vi "Begin.vi"() -> (0 "error out":errorcluster)   [LabVIEW 2013]
doc: "Called before other user functions, this VI is expected to open initial I/O refnums, load in file data, and do all program initialization. Notice that the <B>error out</B> terminal is simply used for data flow. Wiring it to other structures or subVIs ensures that this VI runs first."
uses:
  <vilib>/Rock Robotics/WPI/Joystick/WPI_JoystickDeviceEnum.ctl
  <vilib>/Rock Robotics/SystemInterfaces/Typedef/FPGA_TypedefDigitalModule.ctl
  <vilib>/Rock Robotics/SystemInterfaces/DIO/FPGA_DIOChannel.ctl
  <vilib>/Rock Robotics/SystemInterfaces/DIO/FPGA_DIORelayChannel.ctl
  <vilib>/Rock Robotics/SystemInterfaces/Typedef/FPGA_TypedefSolenoidModule.ctl
  <vilib>/Rock Robotics/WPI/Solenoid/WPI_SolenoidChannel.ctl
  <vilib>/Rock Robotics/WPI/Solenoid/WPI_SolenoidValue.ctl
  <vilib>/Rock Robotics/SystemInterfaces/DIO/FPGA_DIOPWMChannel.ctl
  <vilib>/Rock Robotics/WPI/Encoder/WPI_EncoderType.ctl
  <vilib>/Rock Robotics/WPI/Solenoid/WPI_SolenoidOpenDouble.vi
  <vilib>/Rock Robotics/WPI/Solenoid/WPI_SolenoidSetEnum.vi
  <vilib>/Rock Robotics/WPI/Counter/WPI_CounterDigitalInputToDigitalSource.vi
  <vilib>/Rock Robotics/WPI/RobotDrive/WPI_RobotDriveOpen2MotorWithVictor.vi
  <vilib>/Rock Robotics/WPI/MotorControl/WPI_MotorControlOpen Victor.vi
  <vilib>/Rock Robotics/WPI/Compressor/WPI_CompressorGetSetRefNum.vi
  <vilib>/Rock Robotics/WPI/Camera/WPI_CameraImageSize.ctl
  <vilib>/Rock Robotics/WPI/Camera/WPI_CameraWhite Balance Values.ctl
  <vilib>/Rock Robotics/WPI/Camera/WPI_CameraExposure Values.ctl
  <vilib>/Rock Robotics/WPI/Camera/WPI_CameraFrameRate.ctl
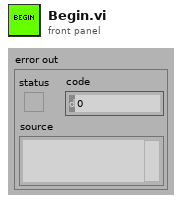
[diagram p1: front panel]
types:
  T1 = typedef "FPGA_DIOChannel.ctl" = enum8{"DIO 1", "DIO 2", "DIO 3", "DIO 4", "DIO 5", "DIO 6", "DIO 7", "DIO 8", "DIO 9", "DIO 10", "DIO 11", "DIO 12", "DIO 13", "DIO 14", "Invalid"}
  T2 = typedef "WPI_SolenoidChannel.ctl" = enum8{"Solenoid 1", "Solenoid 2", "Solenoid 3", "Solenoid 4", "Solenoid 5", "Solenoid 6", "Solenoid 7", "Solenoid 8", "Invalid"}
  T3 = typedef "FPGA_DIOPWMChannel.ctl" = enum8{"PWM 1", "PWM 2", "PWM 3", "PWM 4", "PWM 5", "PWM 6", "PWM 7", "PWM 8", "PWM 9", "PWM 10", "Invalid"}
  T4 = typedef "WPI_EncoderType.ctl" = enum16{"1x", "2x", "4x"}
  T5 = typedef "WPI_SolenoidValue.ctl" = enum16{"Off", "On", "Forward", "Reverse"}
  T6 = typedef "FPGA_TypedefSolenoidModule.ctl" = enum16{"Solenoid Module 1", "Solenoid Module 2"}
  T7 = typedef "FPGA_DIORelayChannel.ctl" = enum8{"Relay 1", "Relay 2", "Relay 3", "Relay 4", "Relay 5", "Relay 6", "Relay 7", "Relay 8", "Invalid"}
  T8 = typedef "WPI_JoystickDeviceEnum.ctl" = enum16{"USB 1", "USB 2", "USB 3", "USB 4", "Kinect 1", "Kinect 2"}
  T9 = typedef "FPGA_TypedefDigitalModule.ctl" = enum16{"Digital Module 1", "Digital Module 2"}
  T10 = typedef "WPI_CameraFrameRate.ctl" = u32
  T11 = typedef "WPI_CameraExposure Values.ctl" = enum16{"Auto", "Flicker-free 50 Hz", "Flicker-free 60 Hz", "Hold current"}
  T12 = typedef "WPI_CameraWhite Balance Values.ctl" = enum16{"Auto", "Fixed indoor", "Fixed outdoor 1", "Fixed outdoor 2", "Fixed fluorescent 1", "Fixed fluorescent 2", "Hold current"}
  T13 = typedef "WPI_CameraImageSize.ctl" = enum16{"640x480", "320x240", "160x120"}
  T14 = typedef "WPI_CameraDevRef.ctl" = cluster{"Camera Address":string, "CameraStatus":errorcluster, "Acquire Image Notifier":refnum<notifier>}
  T15 = typedef "WPI_DigitalInputDevRef.ctl" = cluster{"DevStatus":errorcluster, "DIO Channel":T1, "Digital Module":T9}
  T16 = typedef "WPI_MotorControlDeviceRef.ctl" = cluster{"DeviceStatus":errorcluster, "Type":enum16{"PWM", "CAN"}, "PWM":cluster{"Digital Module":T9, "PWM Channel":T3, "DeadBand":T17}, "CAN":cluster{"Device Number":u8, "Control Mode":T18, "Semaphore":T19, "Max Vout":dbl}, "Invert":bool, "TransformRef":T20, "InvTransformRef":T20}
  T17 = typedef "WPI_PWMDeadband.ctl" = cluster{"Name":string, "maxPositivePwm":i32, "minPositivePwm":i32, "centerPwm":i32, "maxNegativePwm":i32, "minNegativePwm":i32, "angularRange":u16}
  T18 = typedef "WPI_CANJaguar_ControlMode.ctl" = enum8{"Percent VBus", "Current", "Speed", "Position", "Voltage"}
  T19 = typedef "Semaphore RefNum" = refnum<k1>
  T20 = typedef "WPI_PWMTransform_ConPane.ctl" = refnum<vi>
  T21 = typedef "WPI_SolenoidDevRef.ctl" = cluster{"DevStatus":errorcluster, "Solenoid Module":T6, "Forward Solenoid Channel":T2, "Reverse Solenoid Channel":T2}
  T22 = typedef "FPGA_CounterEncoderSourceConvertionLVSourceType.ctl" = cluster{"DevStatus":errorcluster, "AnalogTriggerMode?":bool, "DigitalMode":cluster{"Digital Module":T9, "DIO Channel":T23}, "AnalogTriggerMode":cluster{"AnalogTriggerIndex":T24, "OutputType":T25}}
  T23 = typedef "FPGA_DIODigitalSourceChannel.ctl" = enum8{"DIO 1", "DIO 2", "DIO 3", "DIO 4", "DIO 5", "DIO 6", "DIO 7", "DIO 8", "DIO 9", "DIO 10", "DIO 11", "DIO 12", "DIO 13", "DIO 14", "Disabled"}
  T24 = typedef "FPGA_AnalogTriggerIndex.ctl" = enum8{"Trig 0", "Trig 1", "Trig 2", "Trig 3", "Trig 4", "Trig 5", "Trig 6", "Trig 7", "Invalid"}
  T25 = typedef "FPGA_AnalogTriggerOutType.ctl" = enum16{"InWindow", "TriggerState", "Rising", "Falling"}
  T26 = typedef "WPI_CompressorDevRef.ctl" = cluster{"DevStatus":errorcluster, "DigitalInputDevRef":T15, "RelayDevRef":T27}
  T27 = typedef "WPI_RelayDevRef.ctl" = cluster{"DevStatus":errorcluster, "Relay Channel":T7, "Digital Module":T9, "Relay Direction":T28}
  T28 = typedef "WPI_RelayDirection.ctl" = enum16{"Both directions", "Forward only", "Reverse only"}
  T29 = typedef "WPI_RobotDriveDevRef.ctl" = cluster{"DevStatus":errorcluster, "Motors[]":T16[], "Square Inputs":bool, "Max Output":dbl, "Isochronous":bool}
  T30 = typedef "WPI_EncoderDevRef.ctl" = cluster{"DevStatus":errorcluster, "EncoderIndex":T31, "CounterIndex":T32, "DistancePerCount":dbl, "Decoding Type":T4}
  T31 = typedef "FPGA_EncoderIdx.ctl" = enum8{"Enc 0", "Enc 1", "Enc 2", "Enc 3", "Invalid"}
  T32 = typedef "FPGA_CounterCtrSystemIndex.ctl" = enum8{"Ctr 0", "Ctr 1", "Ctr 2", "Ctr 3", "Ctr 4", "Ctr 5", "Ctr 6", "Ctr 7", "Invalid"}
  T33 = typedef "WPI_JoystickDevRef.ctl" = cluster{"Device":T8}
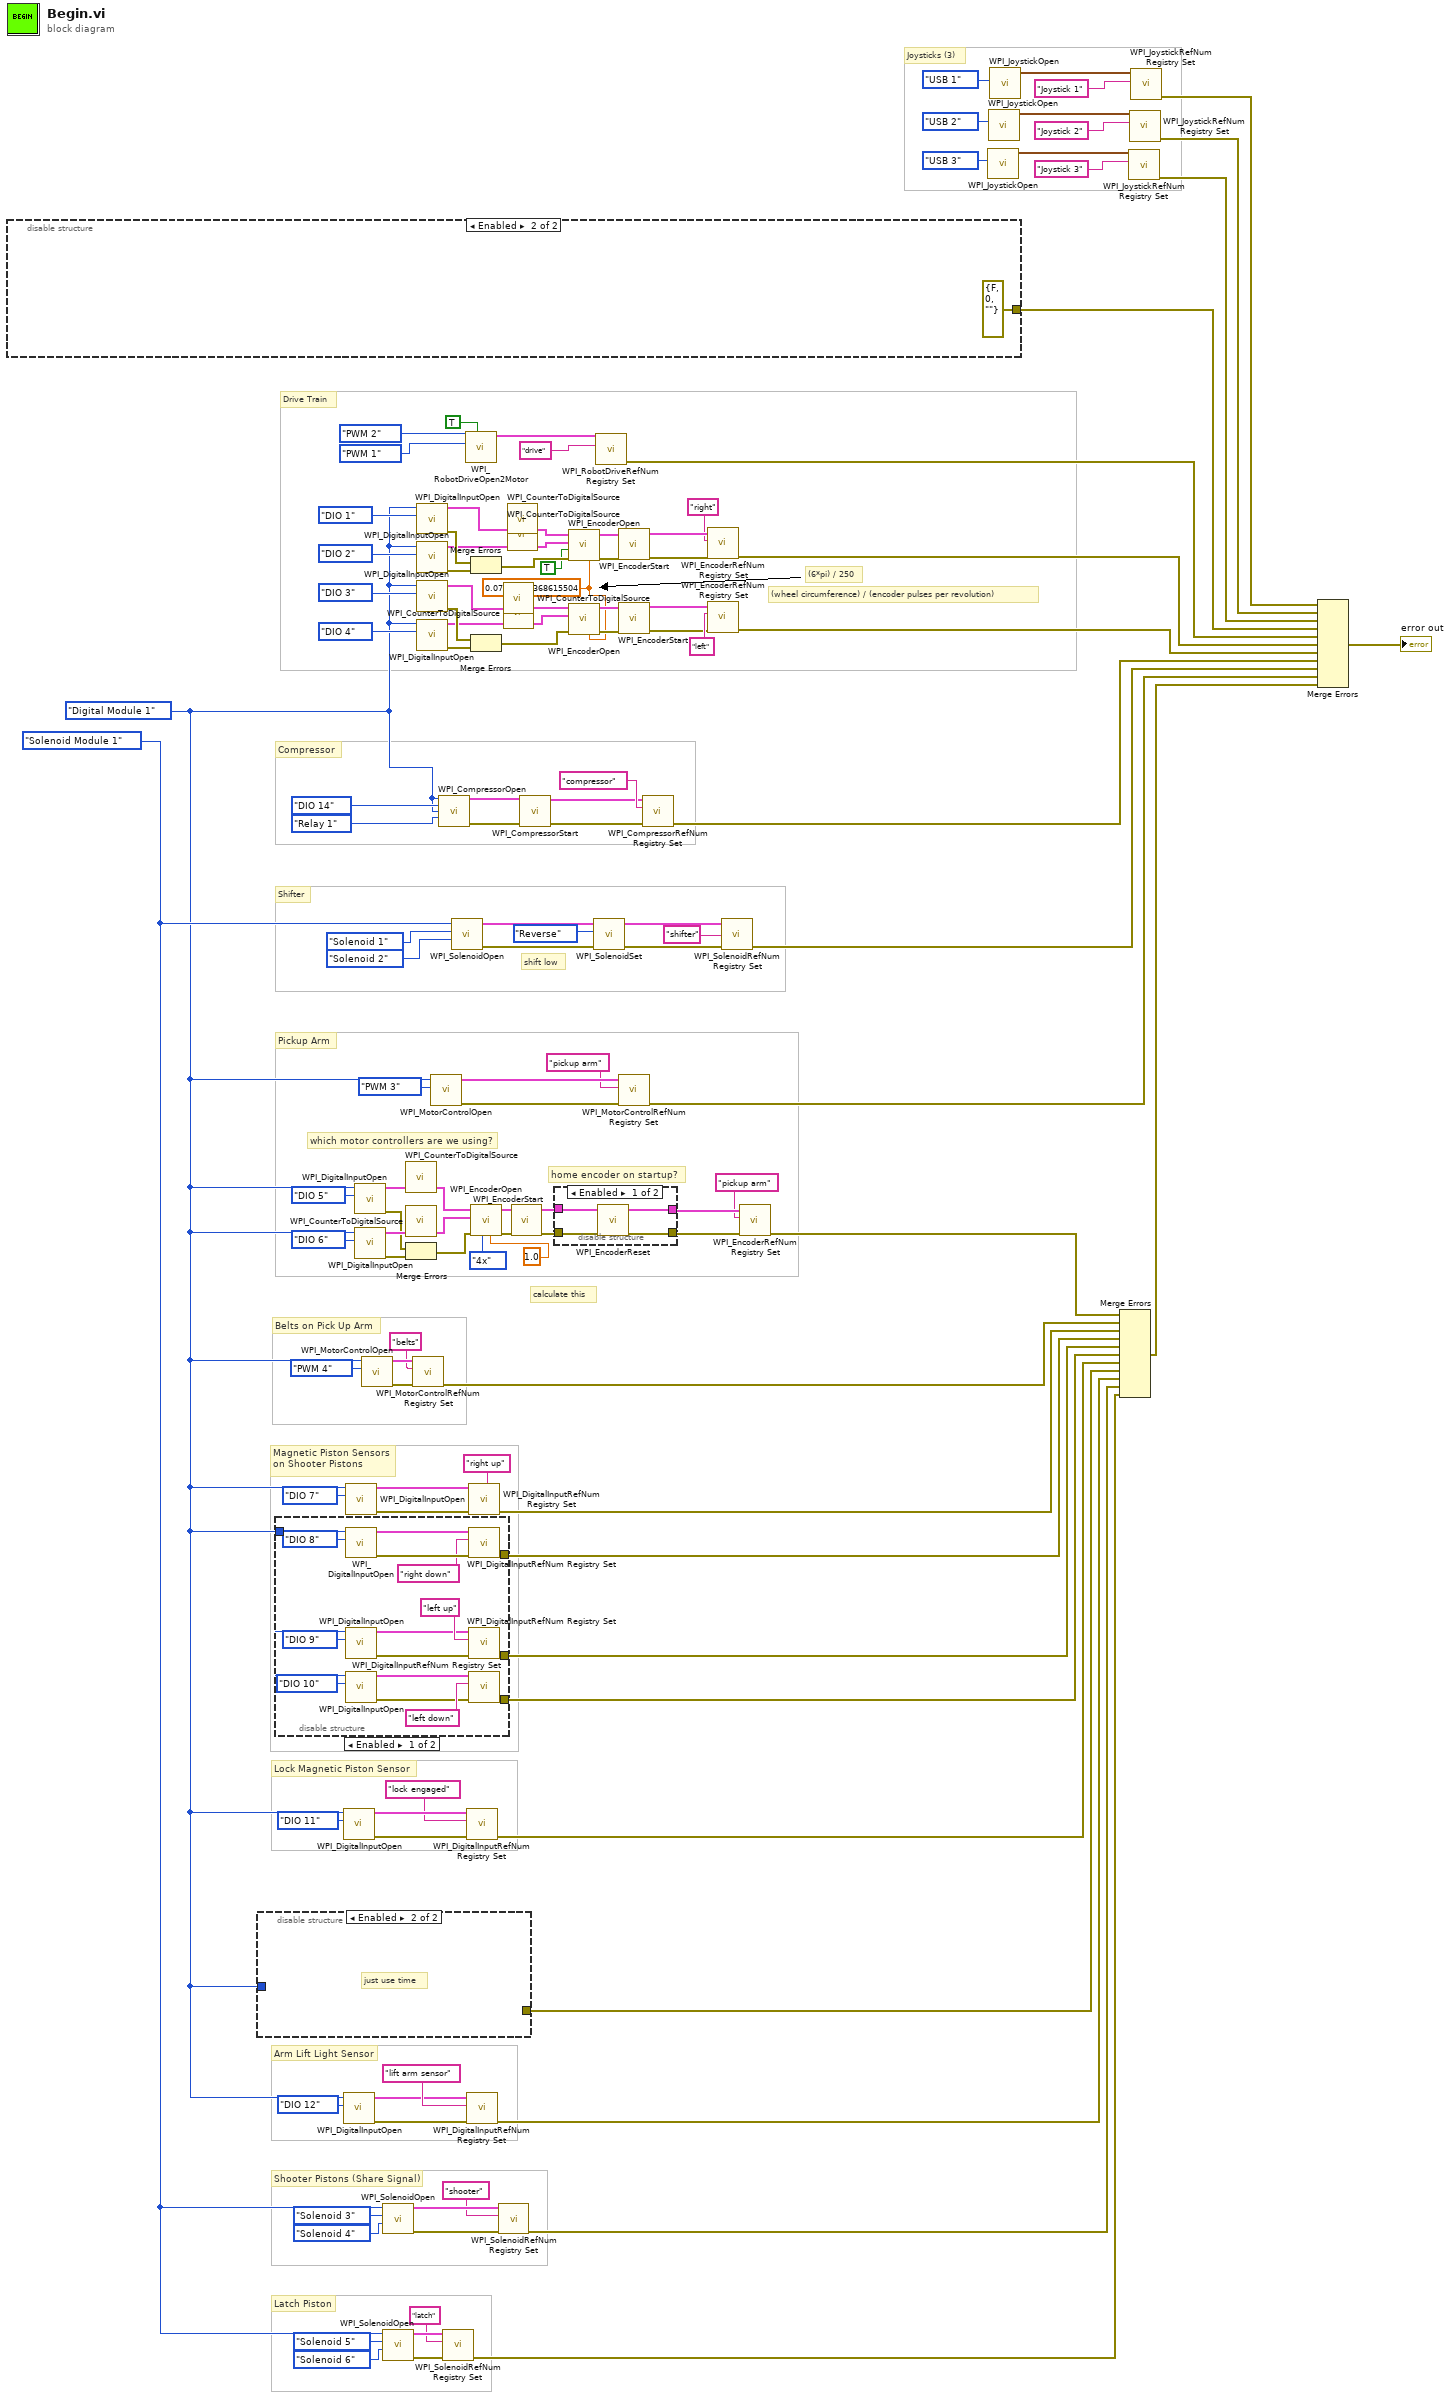
[diagram p0: block diagram]
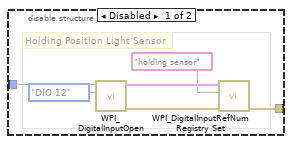
[diagram p3: hidden frame]
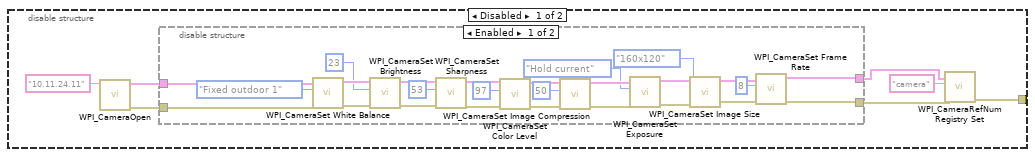
[diagram p5: hidden frame]
diagram:
  w76 = 0.07539822368615504 ("DistancePerCount")
  w17 = FPGA_TypedefSolenoidModule."Solenoid Module 1" ("Solenoid Module (Module 1)")
  w6 = FPGA_TypedefDigitalModule."Digital Module 1" ("Digital Module (Module 1)")
  # "Lock Magnetic Piston Sensor"
  # "Arm Lift Light Sensor"
  # "Joysticks (3)"
  # "Latch Piston"
  # "Shooter Pistons (Share Signal)"
  # "Magnetic Piston Sensors\non Shooter Pistons"
  # "Belts on Pick Up Arm"
  # "calculate this"
  # "Pickup Arm"
  # "home encoder on startup?"
  # "Shifter"
  # "Compressor"
  # "Drive Train"
  # "which motor controllers are we using?"
  # "shift low"
  # "(wheel circumference) / (encoder pulses per revolution)"
  # "(6*pi) / 250"
  n1 = disable-structure shown="Enabled" {
    disable-tunnel: [w133 errorcluster {"status"=FALSE, "code"=0, "source"=""} ("error out")] -> w120
    frame Disabled {
      n2 = call <vilib>:"WPI_CameraOpen.vi"("Camera Address"="10.11.24.11") -> ("error out"=w135:errorcluster, "CameraDevRef"=w137:T14)  [unwired: 9 in]
      n3 = disable-structure shown="Enabled" {
        disable-tunnel: w137 -> [w163 w167]
        disable-tunnel: [w141 w167] -> w136
        disable-tunnel: w135 -> [w150 w166]
        disable-tunnel: [w140 w166] -> w134
        frame Enabled {
          n4 = call <vilib>:"WPI_CameraSet White Balance.vi"("error in (no error)"=w150, "White Balance"=WPI_CameraWhite_Balance_Values."Fixed outdoor 1", "CameraDevRef"=w163) -> ("error out"=w151:errorcluster, "CameraDevRef Out"=w162:T14)  [unwired: 7 in]
          n5 = call <vilib>:"WPI_CameraSet Brightness.vi"("error in (no error)"=w151, "Brightness"=23, "CameraDevRef"=w162) -> ("error out"=w152:errorcluster, "CameraDevRef Out"=w161:T14)  [unwired: 7 in]
          n6 = call <vilib>:"WPI_CameraSet Sharpness.vi"("error in (no error)"=w152, "Sharpness"=53, "CameraDevRef"=w161) -> ("error out"=w153:errorcluster, "CameraDevRef Out"=w160:T14)  [unwired: 7 in]
          n7 = call <vilib>:"WPI_CameraSet Color Level.vi"("error in (no error)"=w153, "Color Level"=97, "CameraDevRef"=w160) -> ("error out"=w154:errorcluster, "CameraDevRef Out"=w159:T14)  [unwired: 7 in]
          n8 = call <vilib>:"WPI_CameraSet Image Compression.vi"("error in (no error)"=w154, "Compression"=50, "CameraDevRef"=w159) -> ("error out"=w165:errorcluster, "CameraDevRef Out"=w164:T14)  [unwired: 7 in]
          n9 = call <vilib>:"WPI_CameraSet Exposure.vi"("error in (no error)"=w165, "Exposure"=WPI_CameraExposure_Values."Hold current", "CameraDevRef"=w164) -> ("error out"=w155:errorcluster, "CameraDevRef Out"=w158:T14)  [unwired: 7 in]
          n10 = call <vilib>:"WPI_CameraSet Image Size.vi"("error in (no error)"=w155, "Image Size"=WPI_CameraImageSize."160x120", "CameraDevRef"=w158) -> ("error out"=w156:errorcluster, "CameraDevRef Out"=w157:T14)  [unwired: 7 in]
          n11 = call <vilib>:"WPI_CameraSet Frame Rate.vi"("error in (no error)"=w156, "Frame Rate (fps)"=T10 8, "CameraDevRef"=w157) -> ("error out"=w140:errorcluster, "CameraDevRef Out"=w141:T14)  [unwired: 7 in]
        }
        frame Disabled {
        }
      }
      n12 = call <vilib>:"WPI_CameraRefNum Registry Set.vi"("error in (no error)"=w134, "refnum name"="camera", "CameraDevRef"=w136) -> ("error out"=w133:errorcluster)  [unwired: 7 in, 1 out]
    }
    frame Enabled {
    }
  }
  n13 = disable-structure shown="Enabled" {
    disable-tunnel: w6 -> [w170 _]
    disable-tunnel: [w169 _] -> w2
    frame Disabled {
      # "Holding Position Light Sensor"
      n14 = call <vilib>:"WPI_DigitalInputOpen.vi"("DIO Channel"=FPGA_DIOChannel."DIO 12", "Digital Module (Module 1)"=w170) -> ("error out"=w173:errorcluster, "DigitalInputDevRef"=w172:T15)  [unwired: 8 in]
      n15 = call <vilib>:"WPI_DigitalInputRefNum Registry Set.vi"("error in (no error)"=w173, "refnum name"="holding sensor", "DigitalInputDevRef"=w172) -> ("error out"=w169:errorcluster)  [unwired: 7 in, 1 out]
    }
    frame Enabled {
      # "just use time"
    }
  }
  n16 = disable-structure shown="Enabled" {
    disable-tunnel: [w187 _] -> w28
    disable-tunnel: w6 -> [w177 _]
    disable-tunnel: [w176 _] -> w12
    disable-tunnel: [w175 _] -> w11
    frame Enabled {
      n17 = call <vilib>:"WPI_DigitalInputOpen.vi"("DIO Channel"=FPGA_DIOChannel."DIO 8", "Digital Module (Module 1)"=w177) -> ("error out"=w190:errorcluster, "DigitalInputDevRef"=w189:T15)  [unwired: 8 in]
      n18 = call <vilib>:"WPI_DigitalInputOpen.vi"("DIO Channel"=FPGA_DIOChannel."DIO 9", "Digital Module (Module 1)"=w177) -> ("error out"=w178:errorcluster, "DigitalInputDevRef"=w179:T15)  [unwired: 8 in]
      n19 = call <vilib>:"WPI_DigitalInputOpen.vi"("DIO Channel"=FPGA_DIOChannel."DIO 10", "Digital Module (Module 1)"=w177) -> ("error out"=w180:errorcluster, "DigitalInputDevRef"=w181:T15)  [unwired: 8 in]
      n20 = call <vilib>:"WPI_DigitalInputRefNum Registry Set.vi"("error in (no error)"=w190, "refnum name"="right down", "DigitalInputDevRef"=w189) -> ("error out"=w187:errorcluster)  [unwired: 7 in, 1 out]
      n21 = call <vilib>:"WPI_DigitalInputRefNum Registry Set.vi"("error in (no error)"=w178, "refnum name"="left up", "DigitalInputDevRef"=w179) -> ("error out"=w176:errorcluster)  [unwired: 7 in, 1 out]
      n22 = call <vilib>:"WPI_DigitalInputRefNum Registry Set.vi"("error in (no error)"=w180, "refnum name"="left down", "DigitalInputDevRef"=w181) -> ("error out"=w175:errorcluster)  [unwired: 7 in, 1 out]
    }
    frame Disabled {
      # "dang, only one sensor\non the pistons..."
    }
  }
  n23 = call <vilib>:"WPI_DigitalInputOpen.vi"("DIO Channel"=FPGA_DIOChannel."DIO 11", "Digital Module (Module 1)"=w6) -> ("error out"=w9:errorcluster, "DigitalInputDevRef"=w8:T15)  [unwired: 8 in]
  n24 = call <vilib>:"WPI_DigitalInputOpen.vi"("DIO Channel"=FPGA_DIOChannel."DIO 12", "Digital Module (Module 1)"=w6) -> ("error out"=w14:errorcluster, "DigitalInputDevRef"=w15:T15)  [unwired: 8 in]
  n25 = call <vilib>:"WPI_DigitalInputOpen.vi"("DIO Channel"=FPGA_DIOChannel."DIO 7", "Digital Module (Module 1)"=w6) -> ("error out"=w33:errorcluster, "DigitalInputDevRef"=w32:T15)  [unwired: 8 in]
  n26 = call <vilib>:"WPI_DigitalInputOpen.vi"("DIO Channel"=FPGA_DIOChannel."DIO 5", "Digital Module (Module 1)"=w6) -> ("error out"=w51:errorcluster, "DigitalInputDevRef"=w56:T15)  [unwired: 8 in]
  n27 = call <vilib>:"WPI_DigitalInputOpen.vi"("DIO Channel"=FPGA_DIOChannel."DIO 6", "Digital Module (Module 1)"=w6) -> ("error out"=w52:errorcluster, "DigitalInputDevRef"=w55:T15)  [unwired: 8 in]
  n28 = call-poly <vilib>:"WPI_MotorControlOpen.vi"("PWM Channel"=FPGA_DIOPWMChannel."PWM 4", "Digital Module (Module 1)"=w6) -> ("error out"=w39:errorcluster, "MotorControlDeviceRef"=w38:T16)  [unwired: 8 in]
  n29 = call-poly <vilib>:"WPI_SolenoidOpen.vi"("Reverse Solenoid Channel"=WPI_SolenoidChannel."Solenoid 4", "Forward Solenoid Channel"=WPI_SolenoidChannel."Solenoid 3", "Solenoid Module (Module 1)"=w17) -> ("error out"=w23:errorcluster, "SolenoidDevRef"=w22:T21)  [unwired: 7 in]
  n30 = call-poly <vilib>:"WPI_SolenoidOpen.vi"("Reverse Solenoid Channel"=WPI_SolenoidChannel."Solenoid 6", "Forward Solenoid Channel"=WPI_SolenoidChannel."Solenoid 5", "Solenoid Module (Module 1)"=w17) -> ("error out"=w21:errorcluster, "SolenoidDevRef"=w20:T21)  [unwired: 7 in]
  n31 = call-poly <vilib>:"WPI_CounterToDigitalSource.vi"("DigitalInputDevRef"=w56) -> ("Digital Source"=w54:T22)  [unwired: 6 in]
  n32 = call-poly <vilib>:"WPI_CounterToDigitalSource.vi"("DigitalInputDevRef"=w55) -> ("Digital Source"=w53:T22)  [unwired: 6 in]
  n33 = Merge Errors(w51, w52) -> (w50:errorcluster)
  n34 = call <vilib>:"WPI_MotorControlRefNum Registry Set.vi"("error in (no error)"=w39, "refnum name"="belts", "MotorControlDevRef"=w38) -> ("error out"=w36:errorcluster)  [unwired: 7 in, 1 out]
  n35 = call <vilib>:"WPI_DigitalInputOpen.vi"("DIO Channel"=FPGA_DIOChannel."DIO 1", "Digital Module (Module 1)"=w6) -> ("error out"=w70:errorcluster, "DigitalInputDevRef"=w84:T15)  [unwired: 8 in]
  n36 = call <vilib>:"WPI_DigitalInputOpen.vi"("DIO Channel"=FPGA_DIOChannel."DIO 2", "Digital Module (Module 1)"=w6) -> ("error out"=w72:errorcluster, "DigitalInputDevRef"=w69:T15)  [unwired: 8 in]
  n37 = call <vilib>:"WPI_DigitalInputOpen.vi"("DIO Channel"=FPGA_DIOChannel."DIO 3", "Digital Module (Module 1)"=w6) -> ("error out"=w73:errorcluster, "DigitalInputDevRef"=w98:T15)  [unwired: 8 in]
  n38 = call <vilib>:"WPI_DigitalInputOpen.vi"("DIO Channel"=FPGA_DIOChannel."DIO 4", "Digital Module (Module 1)"=w6) -> ("error out"=w75:errorcluster, "DigitalInputDevRef"=w68:T15)  [unwired: 8 in]
  n39 = call-poly <vilib>:"WPI_MotorControlOpen.vi"("PWM Channel"=FPGA_DIOPWMChannel."PWM 3", "Digital Module (Module 1)"=w6) -> ("error out"=w63:errorcluster, "MotorControlDeviceRef"=w62:T16)  [unwired: 8 in]
  n40 = call <vilib>:"WPI_CompressorOpen.vi"("Pressure Switch Digital Module (Module 1)"=w6, "Pressure Switch DIO Channel"=FPGA_DIOChannel."DIO 14", "Relay Digital Module (Module 1)"=w6, "Relay Channel"=FPGA_DIORelayChannel."Relay 1") -> ("CompressorDevRef"=w112:T26, "error out"=w111:errorcluster)  [unwired: 10 in]
  n41 = call <vilib>:"WPI_SolenoidRefNum Registry Set.vi"("error in (no error)"=w21, "refnum name"="latch", "SolenoidDevRef"=w20) -> ("error out"=w5:errorcluster)  [unwired: 7 in, 1 out]
  n42 = call-poly <vilib>:"WPI_SolenoidOpen.vi"("Reverse Solenoid Channel"=WPI_SolenoidChannel."Solenoid 2", "Forward Solenoid Channel"=WPI_SolenoidChannel."Solenoid 1", "Solenoid Module (Module 1)"=w17) -> ("error out"=w103:errorcluster, "SolenoidDevRef"=w104:T21)  [unwired: 7 in]
  n43 = call-poly <vilib>:"WPI_RobotDriveOpen2Motor.vi"("Left Motor Inverted"=TRUE, "Right Motor"=FPGA_DIOPWMChannel."PWM 1", "Left Motor"=FPGA_DIOPWMChannel."PWM 2") -> ("RobotDriveDevRef"=w100:T29)  [unwired: 7 in, 1 out]
  n44 = call <vilib>:"WPI_DigitalInputRefNum Registry Set.vi"("error in (no error)"=w9, "refnum name"="lock engaged", "DigitalInputDevRef"=w8) -> ("error out"=w1:errorcluster)  [unwired: 7 in, 1 out]
  n45 = call <vilib>:"WPI_DigitalInputRefNum Registry Set.vi"("error in (no error)"=w14, "refnum name"="lift arm sensor", "DigitalInputDevRef"=w15) -> ("error out"=w3:errorcluster)  [unwired: 7 in, 1 out]
  n46 = call <vilib>:"WPI_DigitalInputRefNum Registry Set.vi"("error in (no error)"=w33, "refnum name"="right up", "DigitalInputDevRef"=w32) -> ("error out"=w29:errorcluster)  [unwired: 7 in, 1 out]
  n47 = Merge Errors(w70, w72) -> (w71:errorcluster)
  n48 = Merge Errors(w73, w75) -> (w74:errorcluster)
  n49 = call <vilib>:"WPI_EncoderOpen.vi"("DistancePerCount"=1.0, "Decoding Type"=WPI_EncoderType."4x", "error in (no error)"=w50, "BSource"=w53, "ASource"=w54) -> ("error out"=w49:errorcluster, "EncoderDevRef"=w48:T30)  [unwired: 5 in]
  n50 = call <vilib>:"WPI_SolenoidRefNum Registry Set.vi"("error in (no error)"=w23, "refnum name"="shooter", "SolenoidDevRef"=w22) -> ("error out"=w4:errorcluster)  [unwired: 7 in, 1 out]
  n51 = call-poly <vilib>:"WPI_CounterToDigitalSource.vi"("DigitalInputDevRef"=w98) -> ("Digital Source"=w91:T22)  [unwired: 6 in]
  n52 = call-poly <vilib>:"WPI_CounterToDigitalSource.vi"("DigitalInputDevRef"=w68) -> ("Digital Source"=w92:T22)  [unwired: 6 in]
  n53 = call-poly <vilib>:"WPI_CounterToDigitalSource.vi"("DigitalInputDevRef"=w84) -> ("Digital Source"=w90:T22)  [unwired: 6 in]
  n54 = call-poly <vilib>:"WPI_CounterToDigitalSource.vi"("DigitalInputDevRef"=w69) -> ("Digital Source"=w89:T22)  [unwired: 6 in]
  n55 = call <vilib>:"WPI_EncoderStart.vi"("error in (no error)"=w49, "EncoderDevRef"=w48) -> ("error out"=w47:errorcluster, "EncoderDevRef"=w46:T30)  [unwired: 8 in]
  n56 = call <vilib>:"WPI_CompressorStart.vi"("error in (no error)"=w111, "CompressorDevRef"=w112) -> ("error out"=w110:errorcluster, "CompressorDevRef"=w109:T26)  [unwired: 8 in]
  n57 = disable-structure shown="Enabled" {
    disable-tunnel: w47 -> [w194 w195]
    disable-tunnel: w46 -> [w193 w196]
    disable-tunnel: [w192 w196] -> w44
    disable-tunnel: [w191 w195] -> w45
    frame Enabled {
      n58 = call <vilib>:"WPI_EncoderReset.vi"("error in (no error)"=w194, "EncoderDevRef"=w193) -> ("error out"=w191:errorcluster, "EncoderDevRef"=w192:T30)  [unwired: 8 in]
    }
    frame Disabled {
    }
  }
  n59 = call <vilib>:"WPI_EncoderOpen.vi"("DistancePerCount"=w76, "error in (no error)"=w71, "Invert Direction (False)"=TRUE, "BSource"=w89, "ASource"=w90) -> ("error out"=w88:errorcluster, "EncoderDevRef"=w87:T30)  [unwired: 5 in]
  n60 = call <vilib>:"WPI_EncoderOpen.vi"("DistancePerCount"=w76, "error in (no error)"=w74, "BSource"=w92, "ASource"=w91) -> ("error out"=w93:errorcluster, "EncoderDevRef"=w94:T30)  [unwired: 6 in]
  n61 = call-poly <vilib>:"WPI_SolenoidSet.vi"("error in (no error)"=w103, "Value"=WPI_SolenoidValue."Reverse", "SolenoidDevRef"=w104) -> ("error out"=w102:errorcluster, "SolenoidDevRef"=w101:T21)  [unwired: 7 in]
  n62 = call <vilib>:"WPI_RobotDriveRefNum Registry Set.vi"("refnum name"="drive", "RobotDriveDevRef"=w100) -> ("error out"=w119:errorcluster)  [unwired: 8 in, 1 out]
  n63 = call <vilib>:"WPI_EncoderStart.vi"("error in (no error)"=w88, "EncoderDevRef"=w87) -> ("error out"=w86:errorcluster, "EncoderDevRef"=w85:T30)  [unwired: 8 in]
  n64 = call <vilib>:"WPI_EncoderStart.vi"("error in (no error)"=w93, "EncoderDevRef"=w94) -> ("error out"=w95:errorcluster, "EncoderDevRef"=w96:T30)  [unwired: 8 in]
  n65 = call <vilib>:"WPI_MotorControlRefNum Registry Set.vi"("error in (no error)"=w63, "refnum name"="pickup arm", "MotorControlDevRef"=w62) -> ("error out"=w59:errorcluster)  [unwired: 7 in, 1 out]
  n66 = call <vilib>:"WPI_CompressorRefNum Registry Set.vi"("error in (no error)"=w110, "refnum name"="compressor", "CompressorDevRef"=w109) -> ("error out"=w64:errorcluster)  [unwired: 7 in, 1 out]
  n67 = call <vilib>:"WPI_EncoderRefNum Registry Set.vi"("error in (no error)"=w86, "refnum name"="right", "EncoderDevRef"=w85) -> ("error out"=w118:errorcluster)  [unwired: 7 in, 1 out]
  n68 = call <vilib>:"WPI_EncoderRefNum Registry Set.vi"("error in (no error)"=w95, "refnum name"="left", "EncoderDevRef"=w96) -> ("error out"=w117:errorcluster)  [unwired: 7 in, 1 out]
  n69 = call <vilib>:"WPI_SolenoidRefNum Registry Set.vi"("error in (no error)"=w102, "refnum name"="shifter", "SolenoidDevRef"=w101) -> ("error out"=w65:errorcluster)  [unwired: 7 in, 1 out]
  n70 = call <vilib>:"WPI_EncoderRefNum Registry Set.vi"("error in (no error)"=w45, "refnum name"="pickup arm", "EncoderDevRef"=w44) -> ("error out"=w35:errorcluster)  [unwired: 7 in, 1 out]
  n71 = call <vilib>:"WPI_JoystickOpen.vi"("JoystickDevice"=WPI_JoystickDeviceEnum."USB 3") -> ("JoystickDevRef"=w131:T33)  [unwired: 10 in]
  n72 = call <vilib>:"WPI_JoystickOpen.vi"("JoystickDevice"=WPI_JoystickDeviceEnum."USB 2") -> ("JoystickDevRef"=w128:T33)  [unwired: 10 in]
  n73 = call <vilib>:"WPI_JoystickOpen.vi"("JoystickDevice"=WPI_JoystickDeviceEnum."USB 1") -> ("JoystickDevRef"=w125:T33)  [unwired: 10 in]
  n74 = Merge Errors(w35, w36, w29, w28, w12, w11, w1, w2, w3, w4, w5) -> (w34:errorcluster)
  n75 = call <vilib>:"WPI_JoystickRefNum Registry Set.vi"("refnum name"="Joystick 3", "JoystickDevRef"=w131) -> ("error out"=w121:errorcluster)  [unwired: 8 in, 1 out]
  n76 = call <vilib>:"WPI_JoystickRefNum Registry Set.vi"("refnum name"="Joystick 2", "JoystickDevRef"=w128) -> ("error out"=w122:errorcluster)  [unwired: 8 in, 1 out]
  n77 = call <vilib>:"WPI_JoystickRefNum Registry Set.vi"("refnum name"="Joystick 1", "JoystickDevRef"=w125) -> ("error out"=w123:errorcluster)  [unwired: 8 in, 1 out]
  n78 = Merge Errors(w123, w122, w121, w120, w119, w118, w117, w64, w65, w59, w34) -> (→"error out":errorcluster)
